vi "Add RT to RT Message.vi"(4 "create timestamp channel":bool, 6 "parameters":T3(array[cluster]), 7 "number of words":u16=1, 8 "error in":errorcluster, 9 "remote terminals":cluster{"Rx":T4, "Tx":T4}, 10 "name":string, 11 "port in":T1 format="%.0x") -> (0 "error out":errorcluster, 2 "messages":cluster{"Tx":T1, "Rx RT":T1, "Rx BC":T1}={"Tx"=18446744073709551615, "Rx RT"=18446744073709551615, "Rx BC"=18446744073709551615} {"Rx BC" format="%.0x"; "Rx RT" format="%.0x"; "Tx" format="%.0x"}, 3 "port out":T1 format="%.0x")   [LabVIEW 2020, in "AIM MIL-STD-1553 Scripting.lvlib"]
uses:
  AIM MIL-STD-1553 Scripting.lvlib
  Shared/Direction.ctl
  <vilib>/NI VeriStand/Custom Device API/Custom Device Item Ref.ctl
  <vilib>/NI VeriStand/Custom Device API/Custom Device API.lvlib
  Shared/Message Type.ctl
  Shared/Address.ctl
  Shared/Terminal Endpoint.ctl
  Shared/Parameter Definition.ctl
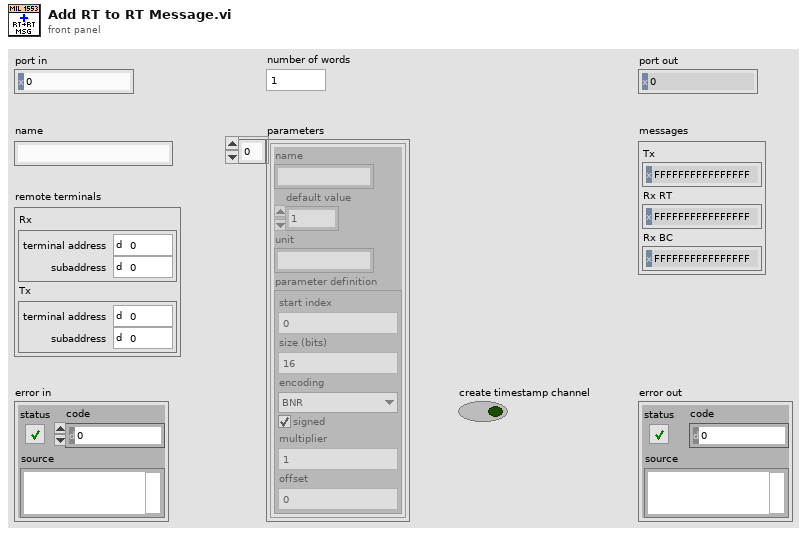
[diagram p1: front panel]
types:
  T1 = typedef "Custom Device API.lvlib/Custom Device Item Ref.ctl" = u64
  T2 = typedef "Parameter Definition.ctl" = cluster{"start index":i32, "size (bits)":i32, "encoding":enum16{"BNR", "BCD", "Discrete"}, "signed":bool, "multiplier":dbl, "offset":dbl}
  T3 = cluster{"name":string, "default value":dbl, "unit":string, "parameter definition":T2}[]
  T4 = typedef "Terminal Endpoint.ctl" = cluster{"terminal address":T5, "subaddress":T5}
  T5 = typedef "Address.ctl" = u16
  T6 = typedef "Direction.ctl" = enum16{"Rx", "Tx"}
  T7 = typedef "Message Type.ctl" = string
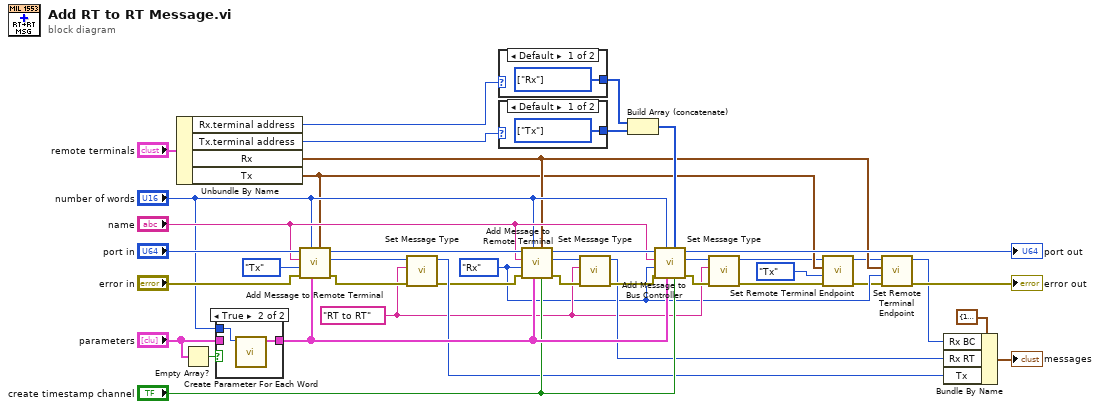
[diagram p0: block diagram]
diagram:
  w17 = T7 "RT to RT" ("message type")
  w10 = Direction."Rx"
  n1 = Unbundle By Name("remote terminals") -> ("Rx.terminal address"=w15:T5, "Tx.terminal address"=w13:T5, "Rx"=w11:T4, "Tx"=w9:T4)
  n2 = Empty Array?(array="parameters") -> (empty?=w41:bool)
  n3 = case shown="True" w41 {
    tunnel: "number of words" -> [_ w44]
    tunnel: "parameters" -> [w42 _]
    tunnel: [w42 w43] -> w31
    frame False {
    }
    frame True {
      n4 = call "Create Parameter For Each Word.vi"("number of words"=w44) -> ("parameters"=w43:T3)  [unwired: 9 in, 1 out]
    }
  }
  n5 = call "Add Message to Remote Terminal.vi"("remote terminal"=w9, "parameters"=w31, "number of words"="number of words", "error in"="error in", "direction"=Direction."Tx", "name"="name", "port in"="port in") -> ("error out"=w25:errorcluster, "message"=w27:T1, "port out"=w37:T1)  [unwired: 2 in]
  n6 = call "Set Message Type.vi"("error in"=w25, "message type"=w17, "message in"=w27) -> ("error out"=w24:errorcluster, "message out"=w26:T1)  [unwired: 7 in]
  n7 = case shown="Default" w15 {
    tunnel: [w45 _] -> w14
    frame Default {
      w45 = enum16{"Rx", "Tx", "Unspecified"}[] [enum."Rx"] items=["Rx", "Tx", "Unspecified"] ("status channels directions")
    }
    frame 31 {
    }
  }
  n8 = case shown="Default" w13 {
    tunnel: [w46 _] -> w12
    frame Default {
      w46 = enum16{"Rx", "Tx", "Unspecified"}[] [enum."Tx"] items=["Rx", "Tx", "Unspecified"] ("status channels directions")
    }
    frame 31 {
    }
  }
  n9 = call "Add Message to Remote Terminal.vi"("create timestamp channel"="create timestamp channel", "remote terminal"=w11, "parameters"=w31, "number of words"="number of words", "error in"=w24, "direction"=w10, "name"="name", "port in"=w37) -> ("error out"=w23:errorcluster, "message"=w21:T1, "port out"=w36:T1)  [unwired: 1 in]
  n10 = call "Set Message Type.vi"("error in"=w23, "message type"=w17, "message in"=w21) -> ("error out"=w22:errorcluster, "message out"=w20:T1)  [unwired: 7 in]
  n11 = Build Array (concatenate)(w14, w12) -> (w16:enum16{"Rx", "Tx", "Unspecified"}[])
  n12 = call "Add Message to Bus Controller.vi"("create timestamp channel"="create timestamp channel", "status channels directions"=w16, "parameters"=w31, "number of words"="number of words", "error in"=w22, "direction"=w10, "name"="name", "port in"=w36) -> ("error out"=w19:errorcluster, "message"=w18:T1, "port out"=→"port out":T1)  [unwired: 1 in]
  n13 = call "Set Message Type.vi"("error in"=w19, "message type"=w17, "message in"=w18) -> ("error out"=w6:errorcluster, "message out"=w7:T1)  [unwired: 7 in]
  n14 = call "Set Remote Terminal Endpoint.vi"("error in"=w6, "direction"=Direction."Tx", "remote terminal"=w9, "message in"=w7) -> ("error out"=w3:errorcluster, "message out"=w4:T1)  [unwired: 6 in]
  n15 = call "Set Remote Terminal Endpoint.vi"("error in"=w3, "direction"=w10, "remote terminal"=w11, "message in"=w4) -> ("error out"=→"error out":errorcluster, "message out"=w1:T1)  [unwired: 6 in]
  n16 = Bundle By Name(cluster=cluster{"Tx":T1, "Rx RT":T1, "Rx BC":T1} {"Tx"=18446744073709551615, "Rx RT"=18446744073709551615, "Rx BC"=18446744073709551615} ("messages"), "Rx BC"=w1, "Rx RT"=w20, "Tx"=w26) -> (→"messages":cluster{"Tx":T1, "Rx RT":T1, "Rx BC":T1})
